vi "MAIN.vi"() -> ()   [LabVIEW 2017]
uses:
  <vilib>/vision/NI_Vision_Development_Module.lvlib
panel:
  out "错误输出":errorcluster
  out "Image Out 2":T1(plugin-control)
  out "输出簇":T2 {"Rotation" format="%.2f"; "Left" scale=0.0..1024.0; "Right" scale=0.0..1024.0}
  in  "Rectangle 3":T2 {"Rotation" min=-90.0 max=90.0 step=1.0 format="%.2f"; "Left" scale=0.0..1024.0; "Right" scale=0.0..1024.0}
  in  "Rectangle 2":T2 {"Rotation" min=-90.0 max=90.0 step=1.0 format="%.2f"; "Left" scale=0.0..1024.0; "Right" scale=0.0..1024.0}
  out "车牌号":string
  in  "Rectangle":T2 {"Rotation" min=-90.0 max=90.0 step=1.0 format="%.2f"; "Left" scale=0.0..1024.0; "Right" scale=0.0..1024.0}
  out "定位车牌":T1(plugin-control)
  out "Caliper Results (Caliper 1)":sgl[][](array[numeric]) format="%.2f"
  out "Image":T1(plugin-control)
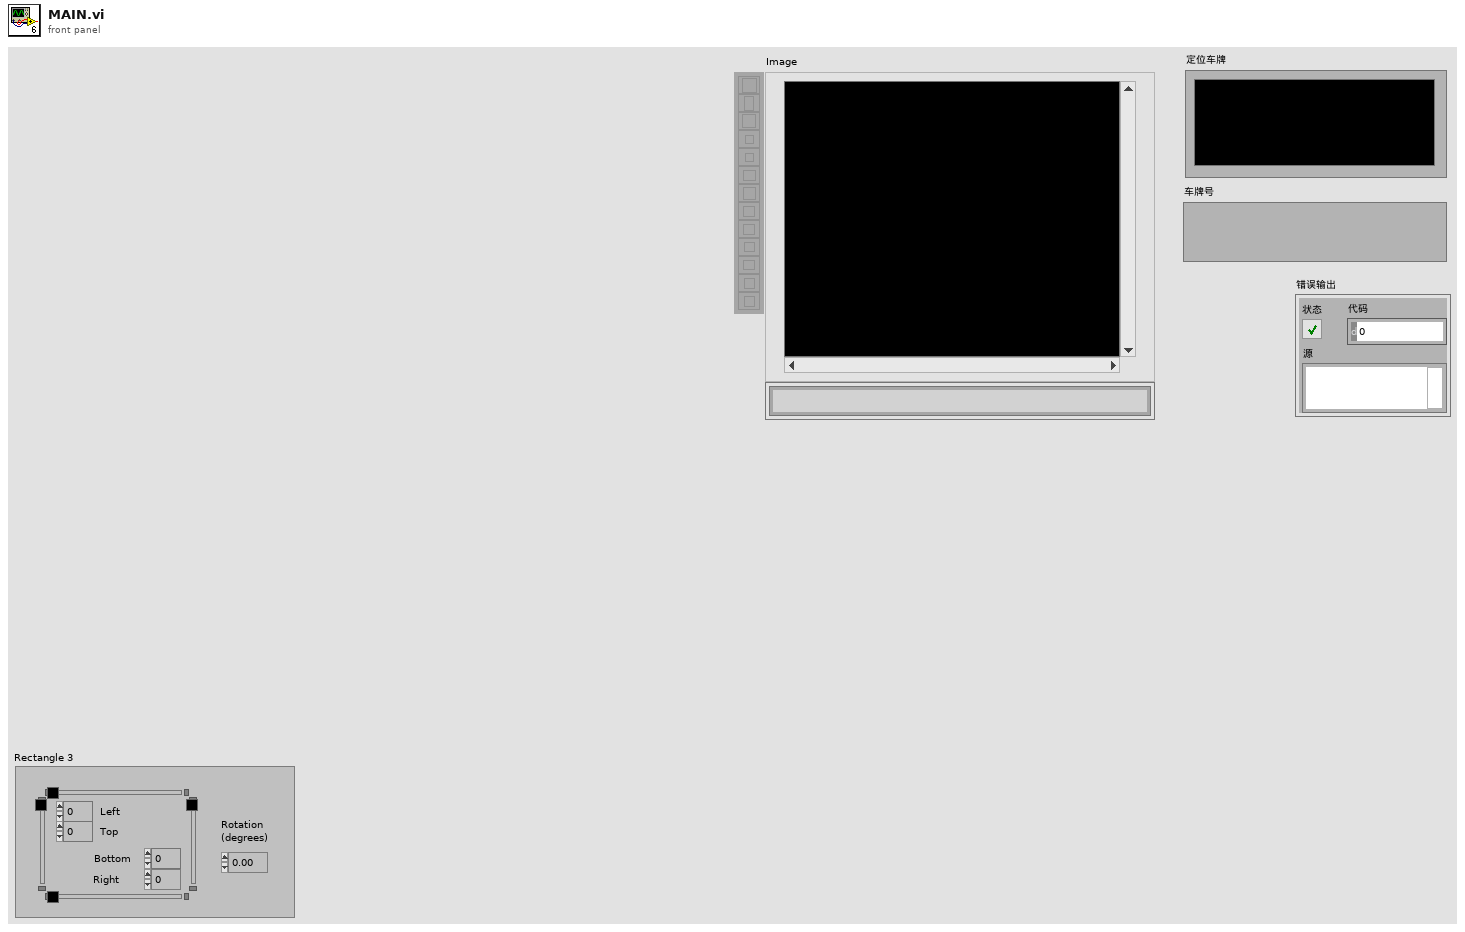
[diagram p1: front panel]
types:
  T1 = typedef "IMAQ Image.ctl" = refnum<image>
  T2 = typedef "IMAQ Rectangle" = cluster{"Left":i32, "Top":i32, "Right":i32, "Bottom":i32, "Rotation":dbl}
  T3 = typedef "Image Type" = u32
  T4 = cluster{"Left":i32, "Top":i32, "Right":i32, "Bottom":i32}
  T5 = typedef "ROI Descriptor" = cluster{"Global Rectangle":i32[], "Contours":cluster{"ID":enum32{"External", "Internal"}, "Type":u32, "Coordinates":i32[]}[]}
  T6 = cluster{"Pixels ":cluster{"Start":cluster{"X":dbl, "Y":dbl}, "End":cluster{"X":dbl, "Y":dbl}}, "Real World":cluster{"Start":cluster{"X":dbl, "Y":dbl}, "End":cluster{"X":dbl, "Y":dbl}}}
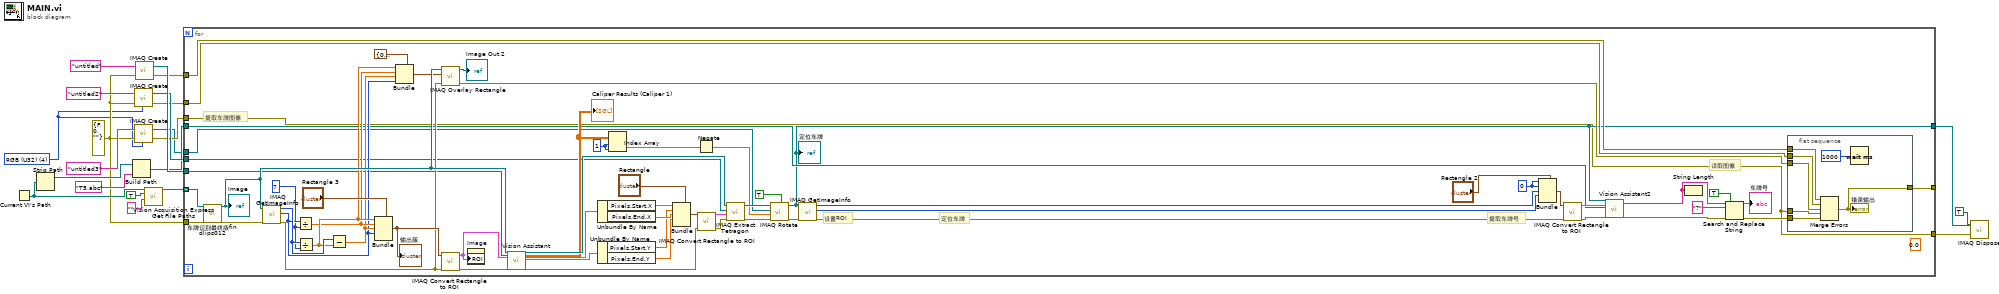
[diagram p0: block diagram]
diagram:
  w4 = T3 4 items=["Grayscale (U8)", "Grayscale (I16)", "Grayscale (SGL)", "Complex (CSG)", "RGB (U32)", "HSL (U32)", "RGB (U64)", "Grayscale (U16)"] ("Image Type")
  w7 = errorcluster {"status"=FALSE, "code"=0, "source"=""} ("error in (no error)")
  n1 = Current VI's Path() -> (path=w9:path)
  n2 = Strip Path(path=w9) -> (stripped path=w18:path)  [unwired: 1 out]
  n3 = Build Path(base path=w18, name or relative path="T5.abc" ("名称或相对路径")) -> (appended path=w11:path)
  n4 = call "IMAQ Create"("Image Name"="untitled2", "Image Type"=w4, "error in (no error)"=w7) -> ("New Image"=w14:T1, "error out"=w12:errorcluster)  [unwired: 2 in]
  n5 = call "IMAQ Create"("Image Name"="untitled3", "Image Type"=w4, "error in (no error)"=w7) -> ("New Image"=w5:T1, "error out"=w6:errorcluster)  [unwired: 2 in]
  n6 = call "IMAQ Create"("Image Name"="untitled", "error in (no error)"=w7) -> ("New Image"=w16:T1, "error out"=w13:errorcluster)  [unwired: 3 in]
  n7 = call <vilib>:"Vision Acquisition Express Get File Paths.vi"("Image File Type (All Types)"="", "Cycle Through Folder"=TRUE, "File Path"=w9) -> ("File Paths"=w20:path[])  [unwired: 8 out]
  n8 = for {
    tunnel: w20 -> [w36] mode=indexing
    tunnel: w16 -> [w35]
    tunnel: w7 -> [w34]
    tunnel: w14 -> [w33]
    tunnel: w13 -> [w32]
    tunnel: w12 -> [w31]
    tunnel: w11 -> [w30]
    tunnel: w6 -> [w22]
    tunnel: w5 -> [w27]
    tunnel: [w25] -> _
    tunnel: [w22] -> w3
    tunnel: [w23] -> w2
    w56 = 1 ("index (row)")
    w26 = 7 ("y")
    (unwired) sgl 0.0 ("Replace Value")
    w29 = 0 ("Left")
    # "提取车牌号"
    # "提取车牌图像"
    # "定位车牌"
    # "设置ROI"
    # "读取图像"
    n9 = call "车牌识别最终版findlips012.vi"("Image Path"=w36, "error in"=w34) -> ("Image Out"=w66:T1, "error out"=w28:errorcluster)  [unwired: 24 in]
    "Image" <- w66
    n10 = call "IMAQ GetImageInfo"("error in (no error)"=w28, "Image"=w66) -> ("error out"=w46:errorcluster, "Y Resolution"=w57:i32, "X Resolution"=w67:i32)  [unwired: 2 in, 5 out]
    n11 = Divide(x=w57, y=w26) -> (x/y=w62:dbl)
    n12 = Divide(x=w67, y=w26) -> (x/y=w63:dbl)
    n13 = Subtract(x=w67, y=w63) -> (x-y=w61:dbl)
    n14 = Bundle(cluster="Rectangle 3", "Left"=w63, "Top"=w62, "Right"=w61, "Bottom"=w57) -> (w65:T2)  [unwired: 1 in]
    "输出簇" <- w65
    n15 = Bundle(cluster=T4 {"Left"=0, "Top"=0, "Right"=0, "Bottom"=0} ("Rectangle"), "Left"=w63, "Top"=w62, "Right"=w61, "Bottom"=w57) -> (w60:T4)
    n16 = call "IMAQ Overlay Rectangle"("error in (no error)"=w46, "Rectangle"=w60, "Image"=w66) -> ("error out"=w37:errorcluster, "Image Out"=→"Image Out 2":T1)  [unwired: 7 in]
    n17 = call "IMAQ Convert Rectangle to ROI"("error in (no error)"=w46, "Rectangle"=w65) -> ("error out"=w45:errorcluster, "ROI Descriptor"=w59:T5)  [unwired: 7 in]
    n18 = property on="Image" class="ImageControl"("ROI"=w59) -> ()  [unwired: 2 in, 2 out]
    n19 = call "Vision Assistant"("Image In"=w66, "Image Dst"=w35, "ROI Descriptor (Image Mask 1)"=w59, "error in"=w45) -> ("Image Out"=w74:T1, "Caliper Results (Caliper 1)"=w51:sgl[][], "Clamp Points (Max Clamp 1)"=w82:T6, "Clamp Points (Copy of Max Clamp 1)"=w83:T6, "error out"=w44:errorcluster)  [unwired: 19 in]
    "Caliper Results (Caliper 1)" <- w51
    n20 = Unbundle By Name(w82) -> ("Pixels.Start.X"=w79:dbl, "Pixels.End.X"=w78:dbl)
    n21 = Unbundle By Name(w83) -> ("Pixels.Start.Y"=w77:dbl, "Pixels.End.Y"=w76:dbl)
    n22 = Index Array(array=w51, index (row)=w56, index (col)=w56) -> (element=w55:sgl)
    n23 = Bundle(cluster="Rectangle", "Left"=w79, "Top"=w77, "Right"=w78, "Bottom"=w76) -> (w80:T2)  [unwired: 1 in]
    n24 = Negate(x=w55) -> (-x=w52:sgl)
    n25 = call "IMAQ Convert Rectangle to ROI"("error in (no error)"=w44, "Rectangle"=w80) -> ("error out"=w43:errorcluster, "ROI Descriptor"=w75:T5)  [unwired: 7 in]
    n26 = call-poly "IMAQ Extract Tetragon"("error in (no error)"=w43, "ROI Descriptor"=w75, "Image Dst"=w33, "Image Src"=w74) -> ("error out"=w42:errorcluster, "Image Dst Out"=w53:T1)  [unwired: 6 in]
    n27 = call "IMAQ Rotate"("Maintain Size"=TRUE, "error in (no error)"=w42, "Angle (degrees)"=w52, "Image Dst"=w27, "Image Src"=w53) -> ("error out"=w41:errorcluster, "Image Dst Out"=w23:T1)  [unwired: 3 in, 2 out]
    "定位车牌" <- w23
    n28 = call "IMAQ GetImageInfo"("error in (no error)"=w41, "Image"=w23) -> ("error out"=w40:errorcluster, "Y Resolution"=w69:i32, "X Resolution"=w70:i32)  [unwired: 2 in, 5 out]
    n29 = Bundle(cluster="Rectangle 2", "Left"=w29, "Top"=w29, "Right"=w70, "Bottom"=w69) -> (w73:T2)  [unwired: 1 in]
    n30 = call "IMAQ Convert Rectangle to ROI"("error in (no error)"=w40, "Rectangle"=w73) -> ("error out"=w39:errorcluster, "ROI Descriptor"=w71:T5)  [unwired: 7 in]
    n31 = call "Vision Assistant2"("Image In"=w23, "ROI Descriptor (OCR/OCV 1)"=w71, "File Path (OCR/OCV 1)"=w30, "error in"=w39) -> ("String (OCR/OCV 1)"=w50:string, "error out"=w24:errorcluster)  [unwired: 21 in, 1 out]
    n32 = String Length(string=w50) -> ()  [unwired: 1 out]
    n33 = Search and Replace String(replace all?=TRUE ("替换全部？(F)"), input string=w50, search string="?" ("搜索字符串"), error in=w24) -> (result string=→"车牌号":string, error out=w38:errorcluster)  [unwired: 4 in, 2 out]
    n34 = flat-sequence {
      tunnel: w38 -> [w90]
      tunnel: w37 -> [w89]
      tunnel: w32 -> [w88]
      tunnel: w31 -> [w87]
      tunnel: [w85] -> w25
      tunnel: w22 -> [w84]
      frame #0 {
        n35 = Merge Errors(w88, w87, w89, w84, w90) -> (w85:errorcluster)
        "错误输出" <- w85
        n36 = Wait (ms)(milliseconds to wait=u32 1000 ("等待时间（毫秒）")) -> ()  [unwired: 1 out]
      }
    }
  }
  n37 = call "IMAQ Dispose"("All Images? (No)"=TRUE, "Image"=w2, "error in (no error)"=w3) -> ()  [unwired: 3 in, 1 out]
